vi "macro_SimpleMotorFF_Calc_NextV.vi"   [LabVIEW 2019, in "Trajectory_Library.lvlib"]
uses:
  Trajectory_Library.lvlib
types:
  T1 = typedef "Trajectory_Library.lvlib/SIMPLE_MOTOR_FF.ctl" = cluster{"Ks":dbl, "Kv":dbl, "Ka":dbl}
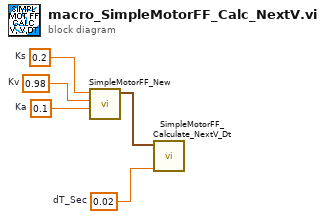
[diagram p0: block diagram]
diagram:
  w1 = 0.02  # dT_Sec
  w3 = 0.2  # Ks
  w4 = 0.98  # Kv
  w5 = 0.1  # Ka
  n1 = call "SimpleMotorFF_New.vi"("Ka"=w5, "Kv"=w4, "Ks"=w3) -> ("SIMPLE_MOTOR_FF"=w2:T1)  [unwired: 8 in]
  n2 = call "SimpleMotorFF_Calculate_NextV_Dt.vi"("dT_Sec"=w1, "SIMPLE_MOTOR_FF"=w2) -> ()  [unwired: 8 in, 2 out]
